vi "exercise example 1.vi"() -> ()   [LabVIEW 2021]
panel:
  in  "Numeric":dbl
  out "indicator":dbl
  in  "y 2":dbl
  in  "x2":dbl
  in  "y1":dbl
  in  "x1":dbl(slide) scale=0.0..10.0
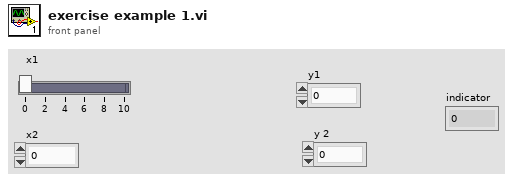
[diagram p1: front panel]
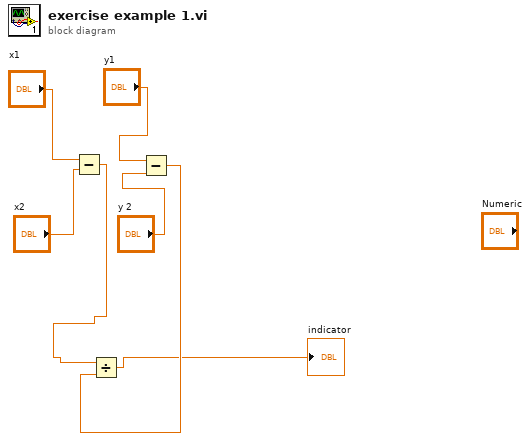
[diagram p0: block diagram]
diagram:
  n1 = Subtract(x="x1", y="x2") -> (x-y=w3:dbl)
  n2 = Subtract(x="y1", y="y 2") -> (x-y=w2:dbl)
  n3 = Divide(x=w3, y=w2) -> (x/y=→"indicator":dbl)
